vi "Lift main.vi"() -> ()   [LabVIEW 2018]
uses:
  <vilib>/Rock Robotics/WPI/ThirdParty/Phoenix-LabVIEW/Motor Controller/Controls/CTRE_Phoenix_MotorControl_FeedbackDevice.ctl
  <vilib>/Rock Robotics/WPI/ThirdParty/Phoenix-LabVIEW/Motor Controller/Controls/CTRE_Phoenix_MotorControl_ControlMode.ctl
  Robot Global Data.vi
  <vilib>/Rock Robotics/WPI/Solenoid/Deprecated/WPI_SolenoidSetBool.vi
  <vilib>/Rock Robotics/WPI/ThirdParty/Phoenix-LabVIEW/Motor Controller/Get/CTRE_Phoenix_MotorController_GetSelectedSensorData.vi
panel:
  in  "Disable?":bool
  in  "Lift Shift":bool
  in  "reset pos":bool
  in  "Setpoint":dbl
  in  "Output":dbl(slide) scale=-1.0..1.0
  in  "Lift Selector":enum16{"Motion Magic", "Manual", "Disable"}(ring)
  in  "PIDF":T1={"P"=2.0, "I"=0.0, "D"=0.0, "F"=0.0, "I zone"=0.0}
  out "Velocity (Raw Sensor Units per 100 ms)":i32
  out "Position (Raw Sensor Units)":i32
  in  "Acceleration":i32=2000
  in  "Cruise Velocity":i32=2000
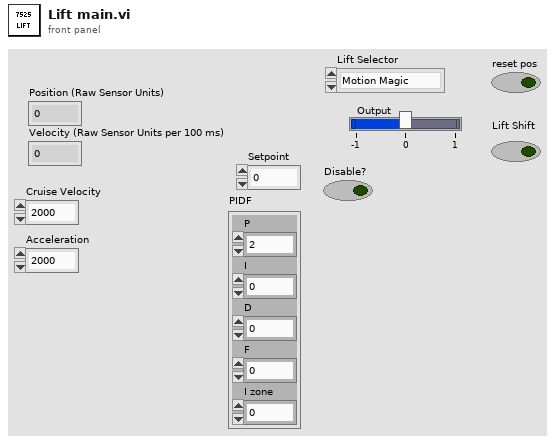
[diagram p1: front panel]
types:
  T1 = cluster{"P":dbl, "I":dbl, "D":dbl, "F":dbl, "I zone":dbl}
  T2 = enum16{"Idle", "Ground", "Hatch Low", "Hatch Mid", "Hatch High", "Cargo Low", "Cargo Mid", "Cargo High", "Cargo Ship", "Cargo Feed"}
  T3 = typedef "CTRE_Phoenix_MotorControl_FeedbackDevice.ctl" = i8
  T4 = typedef "WPI_MotorControlDeviceRef.ctl" = cluster{"DeviceStatus":errorcluster, "Type":T5, "PWM":cluster{"PWM Channel":T6, "DeadBand":T7}, "CAN":cluster{"Device Number":u8, "SetOutput VI Ref":variant, "GetOutput VI Ref":variant, "Enable VI Ref":variant, "Disable VI Ref":variant, "Data":variant}, "Invert":bool, "DIO PWM":cluster{"PWM \"Enable\" Channel":T6, "DIOChannel":T8, "PWM Rate":dbl}}
  T5 = typedef "WPI_MotorControlType.ctl" = enum16{"PWM", "CAN", "DIO PWM"}
  T6 = typedef "FPGA_DIOPWMChannel.ctl" = enum8{"PWM 0", "PWM 1", "PWM 2", "PWM 3", "PWM 4", "PWM 5", "PWM 6", "PWM 7", "PWM 8", "PWM 9", "PWM MXP 0", "PWM MXP 1", "PWM MXP 2", "PWM MXP 3", "PWM MXP 4", "PWM MXP 5", "PWM MXP 6", "PWM MXP 7", "PWM MXP 8", "PWM MXP 9", "Invalid"}
  T7 = typedef "WPI_PWMDeadband.ctl" = cluster{"Name":string, "maxPositivePwm":i32, "minPositivePwm":i32, "centerPwm":i32, "maxNegativePwm":i32, "minNegativePwm":i32, "angularRange":u16}
  T8 = typedef "FPGA_DIOChannel.ctl" = enum8{"DIO 0", "DIO 1", "DIO 2", "DIO 3", "DIO 4", "DIO 5", "DIO 6", "DIO 7", "DIO 8", "DIO 9", "DIO MXP 0", "DIO MXP 1", "DIO MXP 2", "DIO MXP 3", "DIO MXP 4", "DIO MXP 5", "DIO MXP 6", "DIO MXP 7", "DIO MXP 8", "DIO MXP 9", "DIO MXP 10", "DIO MXP 11", "DIO MXP 12", "DIO MXP 13", "DIO MXP 14", "DIO MXP 15", "SPI Port CS1", "SPI Port CS2", "SPI Port CS3", "SPI Port MISO", "SPI Port MOSI", "Invalid"}
  T9 = typedef "WPI_SolenoidDevRef.ctl" = cluster{"DevStatus":errorcluster, "Pneumatics Control Module":u8, "Forward Solenoid Channel":T10, "Reverse Solenoid Channel":T10}
  T10 = typedef "WPI_SolenoidChannel.ctl" = enum8{"Solenoid 0", "Solenoid 1", "Solenoid 2", "Solenoid 3", "Solenoid 4", "Solenoid 5", "Solenoid 6", "Solenoid 7", "Invalid"}
  T11 = typedef "CTRE_Phoenix_MotorControl_ControlMode.ctl" = u16
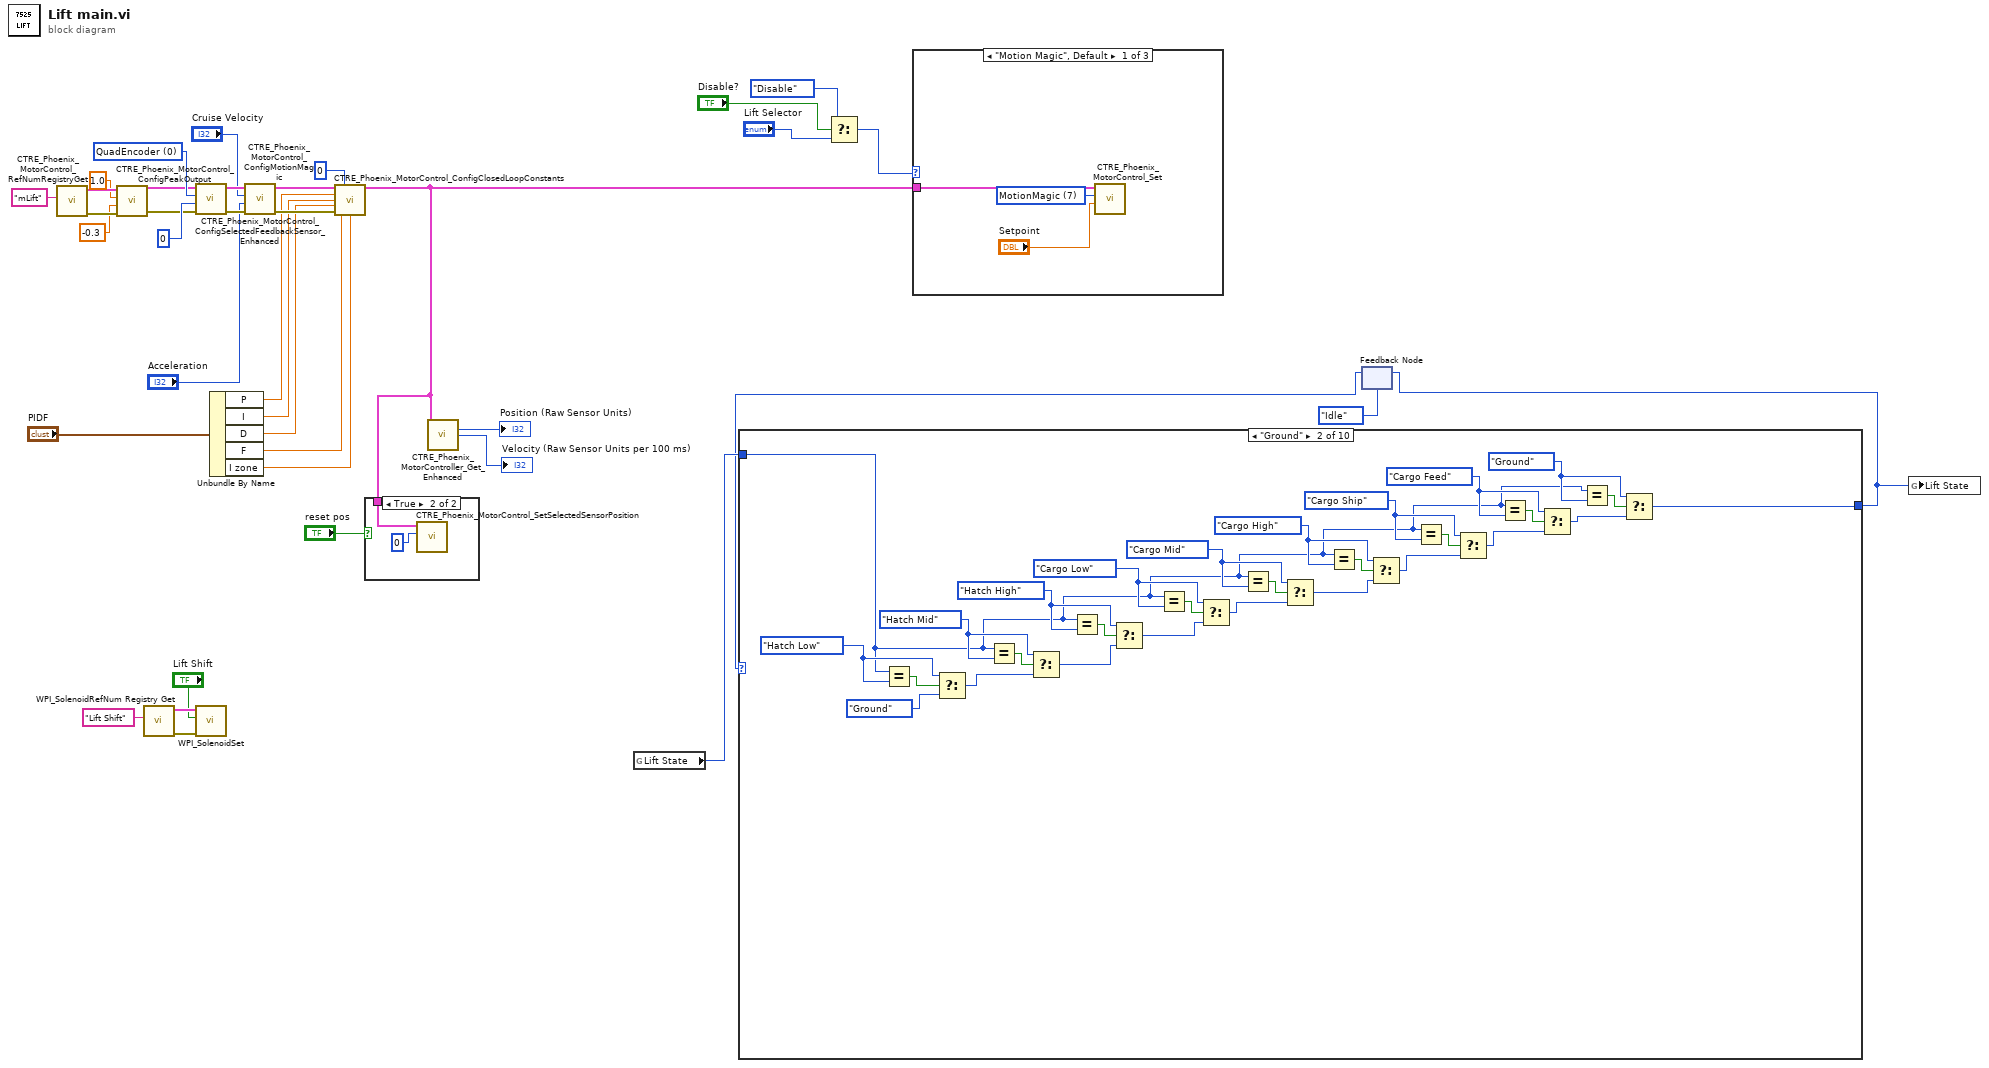
[diagram p0: block diagram]
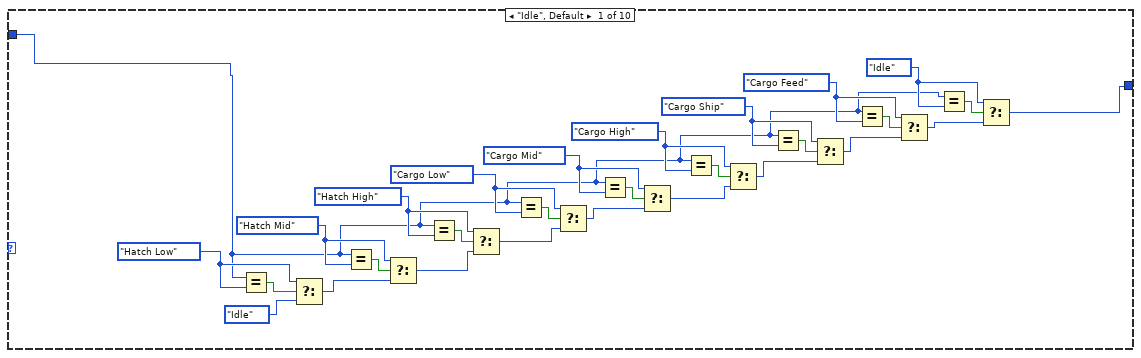
[diagram p2: hidden frame]
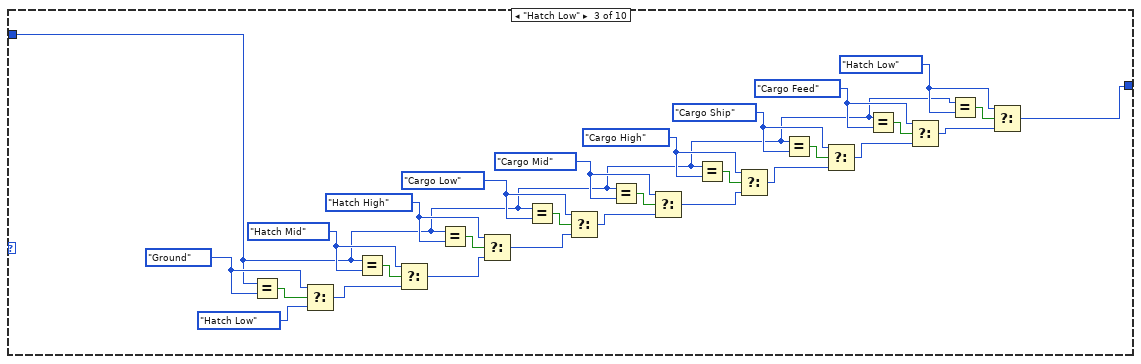
[diagram p3: hidden frame]
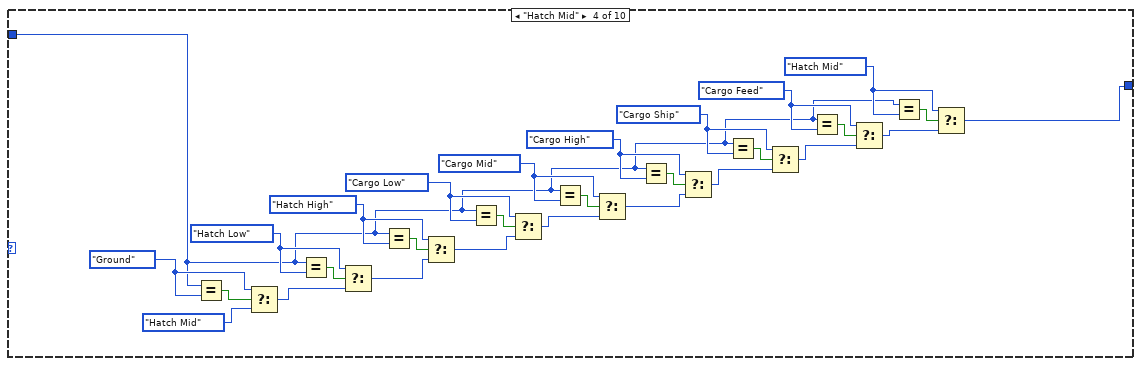
[diagram p4: hidden frame]
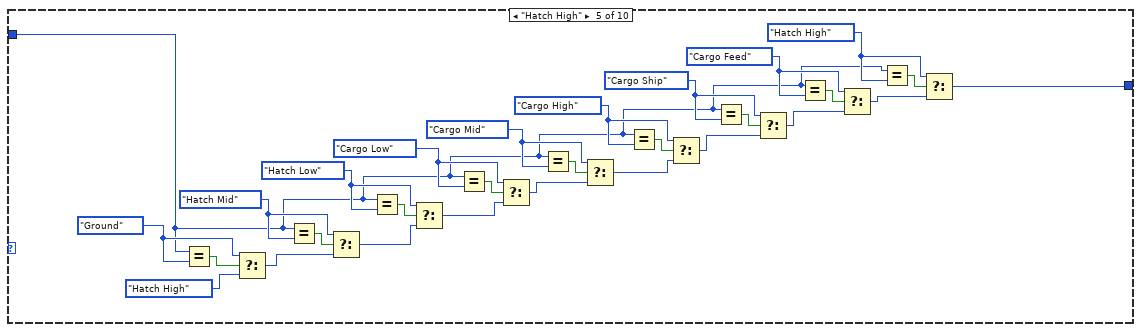
[diagram p5: hidden frame]
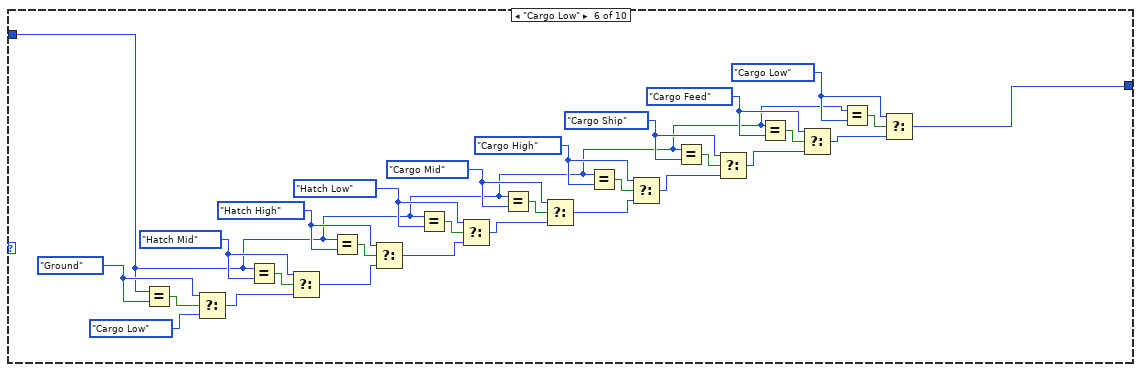
[diagram p6: hidden frame]
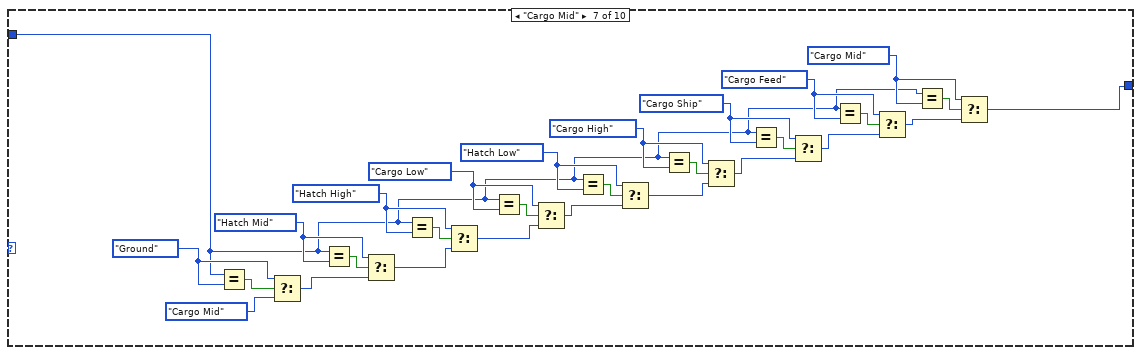
[diagram p7: hidden frame]
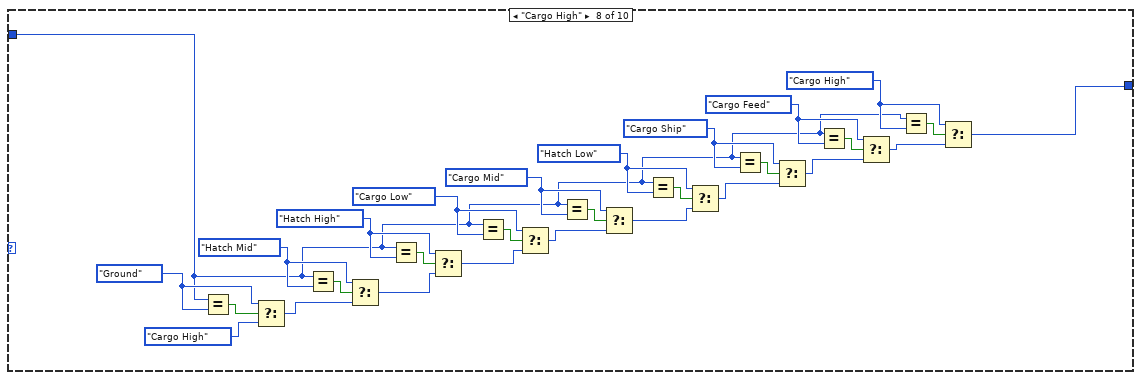
[diagram p8: hidden frame]
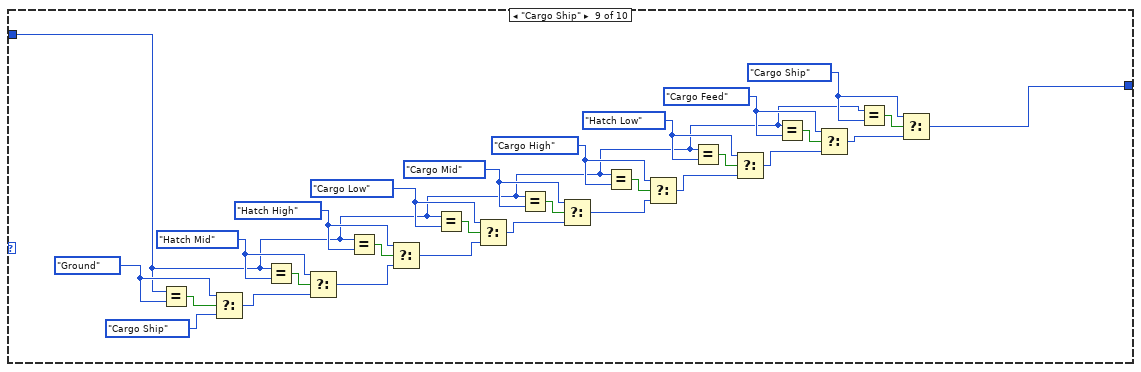
[diagram p9: hidden frame]
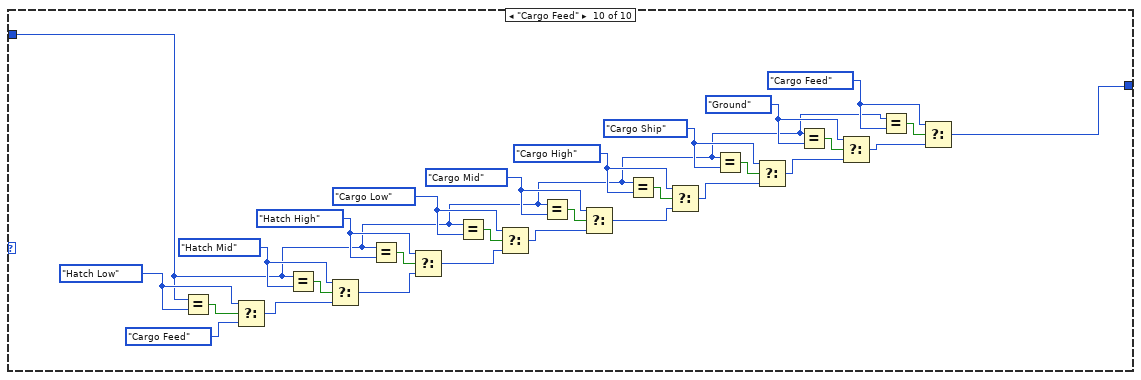
[diagram p10: hidden frame]
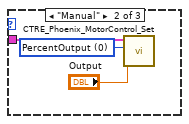
[diagram p12: hidden frame]
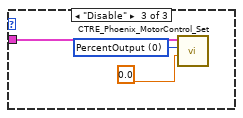
[diagram p13: hidden frame]
diagram:
  w33 = T3 0 items=["QuadEncoder"=0, "Analog"=2, "Tachometer"=4, "Pulse Width Encoded Position"=8, "Sensor Sum (S0 + S1)"=9, "Sensor Difference (D0 - D1)"=10, "Remote Source 0"=11, "Remote Source 1"=12, "Software Emulated"=15] ("Feedback Device")
  n1 = call <vilib>:"CTRE_Phoenix_MotorControl_RefNumRegistryGet.vi"("refnum name"="mLift") -> ("error out"=w37:errorcluster, "PhoenixMotorControlDevRef"=w36:T4)  [unwired: 9 in]
  n2 = call <vilib>:"CTRE_Phoenix_MotorControl_ConfigPeakOutput.vi"("error in (no error)"=w37, "Reverse Peak Percent Output"=-0.3, "Forward Peak Percent Output"=1.0, "PhoenixMotorControlDevRef"=w36) -> ("error out"=w30:errorcluster, "PhoenixMotorControlDevRef"=w31:T4)  [unwired: 6 in]
  n3 = call <vilib>:"WPI_SolenoidRefNum Registry Get.vi"("refnum name"="Lift Shift") -> ("error out"=w12:errorcluster, "SolenoidDevRef"=w11:T9)  [unwired: 9 in]
  n4 = call <vilib>:"CTRE_Phoenix_MotorControl_ConfigSelectedFeedbackSensor_Enhanced.vi"("error in (no error)"=w30, "pidLoopIdx"=0, "Feedback Device"=w33, "PhoenixMotorControlDevRef"=w31) -> ("error out"=w29:errorcluster, "PhoenixMotorControlDevRef"=w28:T4)  [unwired: 6 in]
  n5 = call-poly <vilib>:"WPI_SolenoidSet.vi"("error in (no error)"=w12, "Value"="Lift Shift", "SolenoidDevRef"=w11) -> ()  [unwired: 7 in, 2 out]
  n6 = Unbundle By Name("PIDF") -> ("P"=w19:dbl, "I"=w18:dbl, "D"=w17:dbl, "F"=w16:dbl, "I zone"=w15:dbl)
  n7 = call <vilib>:"CTRE_Phoenix_MotorControl_ConfigMotionMagic.vi"("error in (no error)"=w29, "Acceleration"="Acceleration", "Cruise Velocity"="Cruise Velocity", "PhoenixMotorControlDevRef"=w28) -> ("error out"=w22:errorcluster, "PhoenixMotorControlDevRef"=w23:T4)  [unwired: 6 in]
  n8 = call <vilib>:"CTRE_Phoenix_MotorControl_ConfigClosedLoopConstants.vi"("PhoenixMotorControlDevRef"=w23, "slotIdx"=0, "P"=w19, "I"=w18, "D"=w17, "error in (no error)"=w22, "F"=w16, "I Zone"=w15) -> ("PhoenixMotorControlDevRef"=w14:T4)  [unwired: 6 in, 1 out]
  n9 = case shown="True" "reset pos" {
    tunnel: w14 -> [_ w40]
    frame False {
    }
    frame True {
      n10 = call <vilib>:"CTRE_Phoenix_MotorControl_SetSelectedSensorPosition.vi"("New Sensor Position"=0, "PhoenixMotorControlDevRef"=w40) -> ()  [unwired: 8 in, 2 out]
    }
  }
  n11 = call-poly <vilib>:"CTRE_Phoenix_MotorController_Get_Enhanced.vi"("PhoenixMotorControlDevRef"=w14) -> ("Position (Raw Sensor Units)"=→"Position (Raw Sensor Units)":i32, "Velocity (Raw Sensor Units per 100 ms)"=→"Velocity (Raw Sensor Units per 100 ms)":i32)  [unwired: 11 in, 2 out]
  n12 = global read "Robot Global Data.vi" "Lift State"() -> (w4:T2)
  n13 = Select(t=enum16{"Motion Magic", "Manual", "Disable"}."Disable", s="Disable?", f="Lift Selector") -> (s? t:f=w8:enum16{"Motion Magic", "Manual", "Disable"})
  n14 = case shown="\"Motion Magic\", Default" w8 {
    tunnel: w14 -> [w42 w46 w48]
    frame "Motion Magic", Default {
      w43 = T11 7 items=["PercentOutput"=0, "Position"=1, "Velocity"=2, "Current"=3, "Follower"=5, "MotionProfile"=6, "MotionMagic"=7, "MotionProfileArc"=10, "Disabled"=15] ("Control Mode")
      n15 = call <vilib>:"CTRE_Phoenix_MotorControl_Set.vi"("Output"="Setpoint", "Control Mode"=w43, "PhoenixMotorControlDevRef"=w42) -> ()  [unwired: 7 in, 2 out]
    }
    frame "Manual" {
      w45 = T11 0 items=["PercentOutput"=0, "Position"=1, "Velocity"=2, "Current"=3, "Follower"=5, "MotionProfile"=6, "MotionMagic"=7, "MotionProfileArc"=10, "Disabled"=15] ("Control Mode")
      n16 = call <vilib>:"CTRE_Phoenix_MotorControl_Set.vi"("Output"="Output", "Control Mode"=w45, "PhoenixMotorControlDevRef"=w46) -> ()  [unwired: 7 in, 2 out]
    }
    frame "Disable" {
      w49 = T11 0 items=["PercentOutput"=0, "Position"=1, "Velocity"=2, "Current"=3, "Follower"=5, "MotionProfile"=6, "MotionMagic"=7, "MotionProfileArc"=10, "Disabled"=15] ("Control Mode")
      n17 = call <vilib>:"CTRE_Phoenix_MotorControl_Set.vi"("Output"=0.0, "Control Mode"=w49, "PhoenixMotorControlDevRef"=w48) -> ()  [unwired: 7 in, 2 out]
    }
  }
  n18 = feedback #1(T2."Idle" ("Lift State")) -> (w2:T2)
  n19 = case shown="\"Ground\"" w2 {
    tunnel: w4 -> [w51 w80 w109 w138 w167 w196 w225 w254 w283 w312]
    tunnel: [w50 w79 w108 w137 w166 w195 w224 w253 w282 w311] -> w1
    frame "Idle", Default {
      w54 = T2."Idle" ("Lift State")
      w57 = T2."Cargo Feed" ("Lift State")
      w60 = T2."Cargo Ship" ("Lift State")
      w63 = T2."Cargo High" ("Lift State")
      w66 = T2."Cargo Mid" ("Lift State")
      w69 = T2."Cargo Low" ("Lift State")
      w72 = T2."Hatch High" ("Lift State")
      w75 = T2."Hatch Mid" ("Lift State")
      w76 = T2."Hatch Low" ("Lift State")
      n20 = Equal?(x=w51, y=w76) -> (x = y?=w77:bool)
      n21 = Select(t=w76, s=w77, f=T2."Idle" ("Lift State")) -> (s? t:f=w73:T2)
      n22 = Equal?(x=w51, y=w75) -> (x = y?=w74:bool)
      n23 = Select(t=w75, s=w74, f=w73) -> (s? t:f=w70:T2)
      n24 = Equal?(x=w51, y=w72) -> (x = y?=w71:bool)
      n25 = Select(t=w72, s=w71, f=w70) -> (s? t:f=w67:T2)
      n26 = Equal?(x=w51, y=w69) -> (x = y?=w68:bool)
      n27 = Select(t=w69, s=w68, f=w67) -> (s? t:f=w64:T2)
      n28 = Equal?(x=w51, y=w66) -> (x = y?=w65:bool)
      n29 = Select(t=w66, s=w65, f=w64) -> (s? t:f=w61:T2)
      n30 = Equal?(x=w51, y=w63) -> (x = y?=w62:bool)
      n31 = Select(t=w63, s=w62, f=w61) -> (s? t:f=w58:T2)
      n32 = Equal?(x=w51, y=w60) -> (x = y?=w59:bool)
      n33 = Select(t=w60, s=w59, f=w58) -> (s? t:f=w55:T2)
      n34 = Equal?(x=w51, y=w57) -> (x = y?=w56:bool)
      n35 = Select(t=w57, s=w56, f=w55) -> (s? t:f=w52:T2)
      n36 = Equal?(x=w51, y=w54) -> (x = y?=w53:bool)
      n37 = Select(t=w54, s=w53, f=w52) -> (s? t:f=w50:T2)
    }
    frame "Ground" {
      w83 = T2."Ground" ("Lift State")
      w86 = T2."Cargo Feed" ("Lift State")
      w89 = T2."Cargo Ship" ("Lift State")
      w92 = T2."Cargo High" ("Lift State")
      w95 = T2."Cargo Mid" ("Lift State")
      w98 = T2."Cargo Low" ("Lift State")
      w101 = T2."Hatch High" ("Lift State")
      w104 = T2."Hatch Mid" ("Lift State")
      w105 = T2."Hatch Low" ("Lift State")
      n38 = Equal?(x=w80, y=w105) -> (x = y?=w106:bool)
      n39 = Select(t=w105, s=w106, f=T2."Ground" ("Lift State")) -> (s? t:f=w102:T2)
      n40 = Equal?(x=w80, y=w104) -> (x = y?=w103:bool)
      n41 = Select(t=w104, s=w103, f=w102) -> (s? t:f=w99:T2)
      n42 = Equal?(x=w80, y=w101) -> (x = y?=w100:bool)
      n43 = Select(t=w101, s=w100, f=w99) -> (s? t:f=w96:T2)
      n44 = Equal?(x=w80, y=w98) -> (x = y?=w97:bool)
      n45 = Select(t=w98, s=w97, f=w96) -> (s? t:f=w93:T2)
      n46 = Equal?(x=w80, y=w95) -> (x = y?=w94:bool)
      n47 = Select(t=w95, s=w94, f=w93) -> (s? t:f=w90:T2)
      n48 = Equal?(x=w80, y=w92) -> (x = y?=w91:bool)
      n49 = Select(t=w92, s=w91, f=w90) -> (s? t:f=w87:T2)
      n50 = Equal?(x=w80, y=w89) -> (x = y?=w88:bool)
      n51 = Select(t=w89, s=w88, f=w87) -> (s? t:f=w84:T2)
      n52 = Equal?(x=w80, y=w86) -> (x = y?=w85:bool)
      n53 = Select(t=w86, s=w85, f=w84) -> (s? t:f=w81:T2)
      n54 = Equal?(x=w80, y=w83) -> (x = y?=w82:bool)
      n55 = Select(t=w83, s=w82, f=w81) -> (s? t:f=w79:T2)
    }
    frame "Hatch Low" {
      w112 = T2."Hatch Low" ("Lift State")
      w115 = T2."Cargo Feed" ("Lift State")
      w118 = T2."Cargo Ship" ("Lift State")
      w121 = T2."Cargo High" ("Lift State")
      w124 = T2."Cargo Mid" ("Lift State")
      w127 = T2."Cargo Low" ("Lift State")
      w130 = T2."Hatch High" ("Lift State")
      w133 = T2."Hatch Mid" ("Lift State")
      w134 = T2."Ground" ("Lift State")
      n56 = Equal?(x=w109, y=w134) -> (x = y?=w135:bool)
      n57 = Select(t=w134, s=w135, f=T2."Hatch Low" ("Lift State")) -> (s? t:f=w131:T2)
      n58 = Equal?(x=w109, y=w133) -> (x = y?=w132:bool)
      n59 = Select(t=w133, s=w132, f=w131) -> (s? t:f=w128:T2)
      n60 = Equal?(x=w109, y=w130) -> (x = y?=w129:bool)
      n61 = Select(t=w130, s=w129, f=w128) -> (s? t:f=w125:T2)
      n62 = Equal?(x=w109, y=w127) -> (x = y?=w126:bool)
      n63 = Select(t=w127, s=w126, f=w125) -> (s? t:f=w122:T2)
      n64 = Equal?(x=w109, y=w124) -> (x = y?=w123:bool)
      n65 = Select(t=w124, s=w123, f=w122) -> (s? t:f=w119:T2)
      n66 = Equal?(x=w109, y=w121) -> (x = y?=w120:bool)
      n67 = Select(t=w121, s=w120, f=w119) -> (s? t:f=w116:T2)
      n68 = Equal?(x=w109, y=w118) -> (x = y?=w117:bool)
      n69 = Select(t=w118, s=w117, f=w116) -> (s? t:f=w113:T2)
      n70 = Equal?(x=w109, y=w115) -> (x = y?=w114:bool)
      n71 = Select(t=w115, s=w114, f=w113) -> (s? t:f=w110:T2)
      n72 = Equal?(x=w109, y=w112) -> (x = y?=w111:bool)
      n73 = Select(t=w112, s=w111, f=w110) -> (s? t:f=w108:T2)
    }
    frame "Hatch Mid" {
      w141 = T2."Hatch Mid" ("Lift State")
      w144 = T2."Cargo Feed" ("Lift State")
      w147 = T2."Cargo Ship" ("Lift State")
      w150 = T2."Cargo High" ("Lift State")
      w153 = T2."Cargo Mid" ("Lift State")
      w156 = T2."Cargo Low" ("Lift State")
      w159 = T2."Hatch High" ("Lift State")
      w162 = T2."Hatch Low" ("Lift State")
      w163 = T2."Ground" ("Lift State")
      n74 = Equal?(x=w138, y=w163) -> (x = y?=w164:bool)
      n75 = Select(t=w163, s=w164, f=T2."Hatch Mid" ("Lift State")) -> (s? t:f=w160:T2)
      n76 = Equal?(x=w138, y=w162) -> (x = y?=w161:bool)
      n77 = Select(t=w162, s=w161, f=w160) -> (s? t:f=w157:T2)
      n78 = Equal?(x=w138, y=w159) -> (x = y?=w158:bool)
      n79 = Select(t=w159, s=w158, f=w157) -> (s? t:f=w154:T2)
      n80 = Equal?(x=w138, y=w156) -> (x = y?=w155:bool)
      n81 = Select(t=w156, s=w155, f=w154) -> (s? t:f=w151:T2)
      n82 = Equal?(x=w138, y=w153) -> (x = y?=w152:bool)
      n83 = Select(t=w153, s=w152, f=w151) -> (s? t:f=w148:T2)
      n84 = Equal?(x=w138, y=w150) -> (x = y?=w149:bool)
      n85 = Select(t=w150, s=w149, f=w148) -> (s? t:f=w145:T2)
      n86 = Equal?(x=w138, y=w147) -> (x = y?=w146:bool)
      n87 = Select(t=w147, s=w146, f=w145) -> (s? t:f=w142:T2)
      n88 = Equal?(x=w138, y=w144) -> (x = y?=w143:bool)
      n89 = Select(t=w144, s=w143, f=w142) -> (s? t:f=w139:T2)
      n90 = Equal?(x=w138, y=w141) -> (x = y?=w140:bool)
      n91 = Select(t=w141, s=w140, f=w139) -> (s? t:f=w137:T2)
    }
    frame "Hatch High" {
      w170 = T2."Hatch High" ("Lift State")
      w173 = T2."Cargo Feed" ("Lift State")
      w176 = T2."Cargo Ship" ("Lift State")
      w179 = T2."Cargo High" ("Lift State")
      w182 = T2."Cargo Mid" ("Lift State")
      w185 = T2."Cargo Low" ("Lift State")
      w188 = T2."Hatch Low" ("Lift State")
      w191 = T2."Hatch Mid" ("Lift State")
      w192 = T2."Ground" ("Lift State")
      n92 = Equal?(x=w167, y=w192) -> (x = y?=w193:bool)
      n93 = Select(t=w192, s=w193, f=T2."Hatch High" ("Lift State")) -> (s? t:f=w189:T2)
      n94 = Equal?(x=w167, y=w191) -> (x = y?=w190:bool)
      n95 = Select(t=w191, s=w190, f=w189) -> (s? t:f=w186:T2)
      n96 = Equal?(x=w167, y=w188) -> (x = y?=w187:bool)
      n97 = Select(t=w188, s=w187, f=w186) -> (s? t:f=w183:T2)
      n98 = Equal?(x=w167, y=w185) -> (x = y?=w184:bool)
      n99 = Select(t=w185, s=w184, f=w183) -> (s? t:f=w180:T2)
      n100 = Equal?(x=w167, y=w182) -> (x = y?=w181:bool)
      n101 = Select(t=w182, s=w181, f=w180) -> (s? t:f=w177:T2)
      n102 = Equal?(x=w167, y=w179) -> (x = y?=w178:bool)
      n103 = Select(t=w179, s=w178, f=w177) -> (s? t:f=w174:T2)
      n104 = Equal?(x=w167, y=w176) -> (x = y?=w175:bool)
      n105 = Select(t=w176, s=w175, f=w174) -> (s? t:f=w171:T2)
      n106 = Equal?(x=w167, y=w173) -> (x = y?=w172:bool)
      n107 = Select(t=w173, s=w172, f=w171) -> (s? t:f=w168:T2)
      n108 = Equal?(x=w167, y=w170) -> (x = y?=w169:bool)
      n109 = Select(t=w170, s=w169, f=w168) -> (s? t:f=w166:T2)
    }
    frame "Cargo Low" {
      w199 = T2."Cargo Low" ("Lift State")
      w202 = T2."Cargo Feed" ("Lift State")
      w205 = T2."Cargo Ship" ("Lift State")
      w208 = T2."Cargo High" ("Lift State")
      w211 = T2."Cargo Mid" ("Lift State")
      w214 = T2."Hatch Low" ("Lift State")
      w217 = T2."Hatch High" ("Lift State")
      w220 = T2."Hatch Mid" ("Lift State")
      w221 = T2."Ground" ("Lift State")
      n110 = Equal?(x=w196, y=w221) -> (x = y?=w222:bool)
      n111 = Select(t=w221, s=w222, f=T2."Cargo Low" ("Lift State")) -> (s? t:f=w218:T2)
      n112 = Equal?(x=w196, y=w220) -> (x = y?=w219:bool)
      n113 = Select(t=w220, s=w219, f=w218) -> (s? t:f=w215:T2)
      n114 = Equal?(x=w196, y=w217) -> (x = y?=w216:bool)
      n115 = Select(t=w217, s=w216, f=w215) -> (s? t:f=w212:T2)
      n116 = Equal?(x=w196, y=w214) -> (x = y?=w213:bool)
      n117 = Select(t=w214, s=w213, f=w212) -> (s? t:f=w209:T2)
      n118 = Equal?(x=w196, y=w211) -> (x = y?=w210:bool)
      n119 = Select(t=w211, s=w210, f=w209) -> (s? t:f=w206:T2)
      n120 = Equal?(x=w196, y=w208) -> (x = y?=w207:bool)
      n121 = Select(t=w208, s=w207, f=w206) -> (s? t:f=w203:T2)
      n122 = Equal?(x=w196, y=w205) -> (x = y?=w204:bool)
      n123 = Select(t=w205, s=w204, f=w203) -> (s? t:f=w200:T2)
      n124 = Equal?(x=w196, y=w202) -> (x = y?=w201:bool)
      n125 = Select(t=w202, s=w201, f=w200) -> (s? t:f=w197:T2)
      n126 = Equal?(x=w196, y=w199) -> (x = y?=w198:bool)
      n127 = Select(t=w199, s=w198, f=w197) -> (s? t:f=w195:T2)
    }
    frame "Cargo Mid" {
      w228 = T2."Cargo Mid" ("Lift State")
      w231 = T2."Cargo Feed" ("Lift State")
      w234 = T2."Cargo Ship" ("Lift State")
      w237 = T2."Cargo High" ("Lift State")
      w240 = T2."Hatch Low" ("Lift State")
      w243 = T2."Cargo Low" ("Lift State")
      w246 = T2."Hatch High" ("Lift State")
      w249 = T2."Hatch Mid" ("Lift State")
      w250 = T2."Ground" ("Lift State")
      n128 = Equal?(x=w225, y=w250) -> (x = y?=w251:bool)
      n129 = Select(t=w250, s=w251, f=T2."Cargo Mid" ("Lift State")) -> (s? t:f=w247:T2)
      n130 = Equal?(x=w225, y=w249) -> (x = y?=w248:bool)
      n131 = Select(t=w249, s=w248, f=w247) -> (s? t:f=w244:T2)
      n132 = Equal?(x=w225, y=w246) -> (x = y?=w245:bool)
      n133 = Select(t=w246, s=w245, f=w244) -> (s? t:f=w241:T2)
      n134 = Equal?(x=w225, y=w243) -> (x = y?=w242:bool)
      n135 = Select(t=w243, s=w242, f=w241) -> (s? t:f=w238:T2)
      n136 = Equal?(x=w225, y=w240) -> (x = y?=w239:bool)
      n137 = Select(t=w240, s=w239, f=w238) -> (s? t:f=w235:T2)
      n138 = Equal?(x=w225, y=w237) -> (x = y?=w236:bool)
      n139 = Select(t=w237, s=w236, f=w235) -> (s? t:f=w232:T2)
      n140 = Equal?(x=w225, y=w234) -> (x = y?=w233:bool)
      n141 = Select(t=w234, s=w233, f=w232) -> (s? t:f=w229:T2)
      n142 = Equal?(x=w225, y=w231) -> (x = y?=w230:bool)
      n143 = Select(t=w231, s=w230, f=w229) -> (s? t:f=w226:T2)
      n144 = Equal?(x=w225, y=w228) -> (x = y?=w227:bool)
      n145 = Select(t=w228, s=w227, f=w226) -> (s? t:f=w224:T2)
    }
    frame "Cargo High" {
      w257 = T2."Cargo High" ("Lift State")
      w260 = T2."Cargo Feed" ("Lift State")
      w263 = T2."Cargo Ship" ("Lift State")
      w266 = T2."Hatch Low" ("Lift State")
      w269 = T2."Cargo Mid" ("Lift State")
      w272 = T2."Cargo Low" ("Lift State")
      w275 = T2."Hatch High" ("Lift State")
      w278 = T2."Hatch Mid" ("Lift State")
      w279 = T2."Ground" ("Lift State")
      n146 = Equal?(x=w254, y=w279) -> (x = y?=w280:bool)
      n147 = Select(t=w279, s=w280, f=T2."Cargo High" ("Lift State")) -> (s? t:f=w276:T2)
      n148 = Equal?(x=w254, y=w278) -> (x = y?=w277:bool)
      n149 = Select(t=w278, s=w277, f=w276) -> (s? t:f=w273:T2)
      n150 = Equal?(x=w254, y=w275) -> (x = y?=w274:bool)
      n151 = Select(t=w275, s=w274, f=w273) -> (s? t:f=w270:T2)
      n152 = Equal?(x=w254, y=w272) -> (x = y?=w271:bool)
      n153 = Select(t=w272, s=w271, f=w270) -> (s? t:f=w267:T2)
      n154 = Equal?(x=w254, y=w269) -> (x = y?=w268:bool)
      n155 = Select(t=w269, s=w268, f=w267) -> (s? t:f=w264:T2)
      n156 = Equal?(x=w254, y=w266) -> (x = y?=w265:bool)
      n157 = Select(t=w266, s=w265, f=w264) -> (s? t:f=w261:T2)
      n158 = Equal?(x=w254, y=w263) -> (x = y?=w262:bool)
      n159 = Select(t=w263, s=w262, f=w261) -> (s? t:f=w258:T2)
      n160 = Equal?(x=w254, y=w260) -> (x = y?=w259:bool)
      n161 = Select(t=w260, s=w259, f=w258) -> (s? t:f=w255:T2)
      n162 = Equal?(x=w254, y=w257) -> (x = y?=w256:bool)
      n163 = Select(t=w257, s=w256, f=w255) -> (s? t:f=w253:T2)
    }
    frame "Cargo Ship" {
      w286 = T2."Cargo Ship" ("Lift State")
      w289 = T2."Cargo Feed" ("Lift State")
      w292 = T2."Hatch Low" ("Lift State")
      w295 = T2."Cargo High" ("Lift State")
      w298 = T2."Cargo Mid" ("Lift State")
      w301 = T2."Cargo Low" ("Lift State")
      w304 = T2."Hatch High" ("Lift State")
      w307 = T2."Hatch Mid" ("Lift State")
      w308 = T2."Ground" ("Lift State")
      n164 = Equal?(x=w283, y=w308) -> (x = y?=w309:bool)
      n165 = Select(t=w308, s=w309, f=T2."Cargo Ship" ("Lift State")) -> (s? t:f=w305:T2)
      n166 = Equal?(x=w283, y=w307) -> (x = y?=w306:bool)
      n167 = Select(t=w307, s=w306, f=w305) -> (s? t:f=w302:T2)
      n168 = Equal?(x=w283, y=w304) -> (x = y?=w303:bool)
      n169 = Select(t=w304, s=w303, f=w302) -> (s? t:f=w299:T2)
      n170 = Equal?(x=w283, y=w301) -> (x = y?=w300:bool)
      n171 = Select(t=w301, s=w300, f=w299) -> (s? t:f=w296:T2)
      n172 = Equal?(x=w283, y=w298) -> (x = y?=w297:bool)
      n173 = Select(t=w298, s=w297, f=w296) -> (s? t:f=w293:T2)
      n174 = Equal?(x=w283, y=w295) -> (x = y?=w294:bool)
      n175 = Select(t=w295, s=w294, f=w293) -> (s? t:f=w290:T2)
      n176 = Equal?(x=w283, y=w292) -> (x = y?=w291:bool)
      n177 = Select(t=w292, s=w291, f=w290) -> (s? t:f=w287:T2)
      n178 = Equal?(x=w283, y=w289) -> (x = y?=w288:bool)
      n179 = Select(t=w289, s=w288, f=w287) -> (s? t:f=w284:T2)
      n180 = Equal?(x=w283, y=w286) -> (x = y?=w285:bool)
      n181 = Select(t=w286, s=w285, f=w284) -> (s? t:f=w282:T2)
    }
    frame "Cargo Feed" {
      w315 = T2."Cargo Feed" ("Lift State")
      w318 = T2."Ground" ("Lift State")
      w321 = T2."Cargo Ship" ("Lift State")
      w324 = T2."Cargo High" ("Lift State")
      w327 = T2."Cargo Mid" ("Lift State")
      w330 = T2."Cargo Low" ("Lift State")
      w333 = T2."Hatch High" ("Lift State")
      w336 = T2."Hatch Mid" ("Lift State")
      w337 = T2."Hatch Low" ("Lift State")
      n182 = Equal?(x=w312, y=w337) -> (x = y?=w338:bool)
      n183 = Select(t=w337, s=w338, f=T2."Cargo Feed" ("Lift State")) -> (s? t:f=w334:T2)
      n184 = Equal?(x=w312, y=w336) -> (x = y?=w335:bool)
      n185 = Select(t=w336, s=w335, f=w334) -> (s? t:f=w331:T2)
      n186 = Equal?(x=w312, y=w333) -> (x = y?=w332:bool)
      n187 = Select(t=w333, s=w332, f=w331) -> (s? t:f=w328:T2)
      n188 = Equal?(x=w312, y=w330) -> (x = y?=w329:bool)
      n189 = Select(t=w330, s=w329, f=w328) -> (s? t:f=w325:T2)
      n190 = Equal?(x=w312, y=w327) -> (x = y?=w326:bool)
      n191 = Select(t=w327, s=w326, f=w325) -> (s? t:f=w322:T2)
      n192 = Equal?(x=w312, y=w324) -> (x = y?=w323:bool)
      n193 = Select(t=w324, s=w323, f=w322) -> (s? t:f=w319:T2)
      n194 = Equal?(x=w312, y=w321) -> (x = y?=w320:bool)
      n195 = Select(t=w321, s=w320, f=w319) -> (s? t:f=w316:T2)
      n196 = Equal?(x=w312, y=w318) -> (x = y?=w317:bool)
      n197 = Select(t=w318, s=w317, f=w316) -> (s? t:f=w313:T2)
      n198 = Equal?(x=w312, y=w315) -> (x = y?=w314:bool)
      n199 = Select(t=w315, s=w314, f=w313) -> (s? t:f=w311:T2)
    }
  }
  n200 = feedback-in #1(w1) -> ()
  n201 = global write "Robot Global Data.vi" "Lift State"(w1) -> ()
